vi "VsEP I-O Config.vi"(0 "Params":T1 {"STIMULUS"."dB STEPSIZE" format="%#_3g"; "STIMULUS"."START dB re 1g/ms" step=5}, 9 "Expt State":T6) -> (2 "Expt State out":T6, 3 "Datafile path":path, 4 "Runtime":T5, 6 "hidden out":T3, 10 "Max SPL":dbl, 14 "Analysis":T4, 15 "error out":errorcluster)   [LabVIEW 2020]
uses:
  CFTS Main Panel SubVIs/CFTS-Experiment State.ctl
  Typedefs/VsEP-Runtime Data.ctl
  Typedefs/VsEP-Hidden Params.ctl
  epl-vi-lib/Signal Synthesis VIs/Controls/Gate XCtl/Gate Control.xctl
  Typedefs/VsEP-Analysis State.ctl
  Typedefs/VsEP-Parameters.ctl
  Typedefs/VsEP-Stimulus Control.ctl
  epl-vi-lib/Connection VIs/Type Defs/Input sources.ctl
  epl-vi-lib/Connection VIs/Type Defs/Output sources.ctl
panel:
  out "num SPLs":i32
  in  "error in (no error)":errorcluster
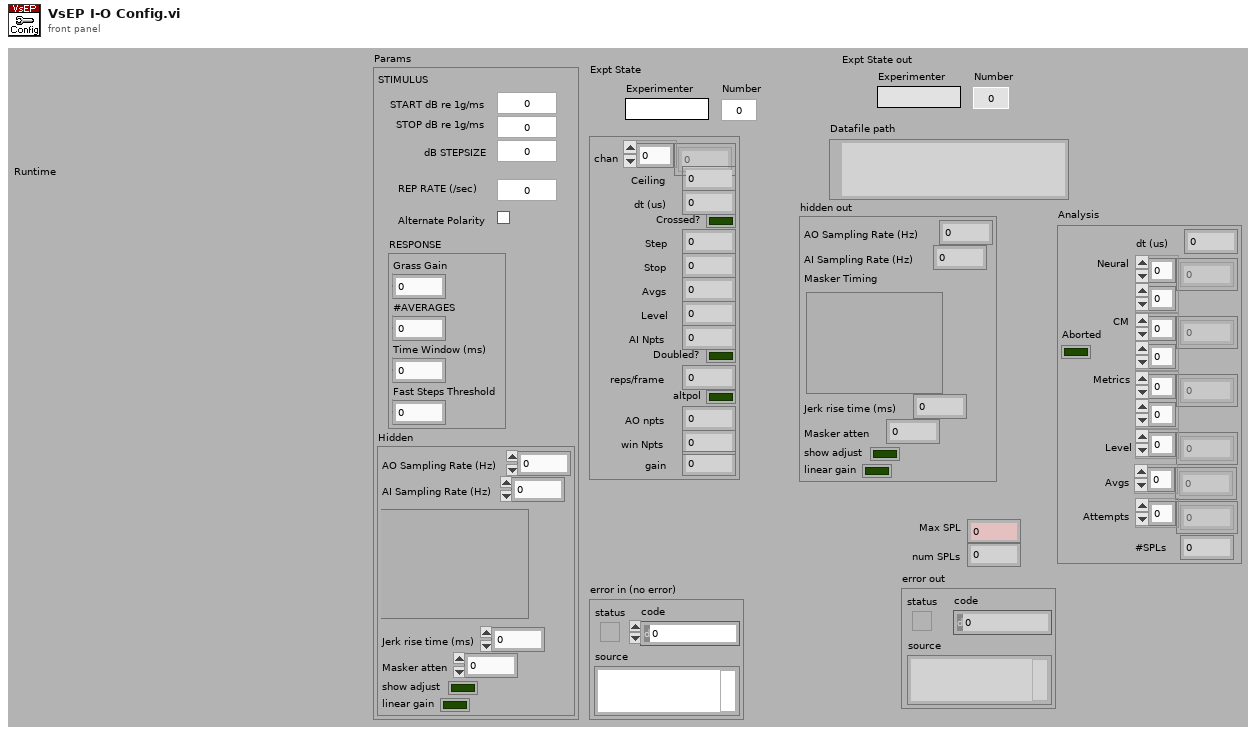
[diagram p1: front panel]
types:
  T1 = typedef "VsEP-Parameters.ctl" = cluster{"STIMULUS":T2, "RESPONSE":cluster{"Grass Gain":i32, "#AVERAGES":i32, "Time Window (ms)":sgl, "Fast Steps Threshold":i32}, "Hidden":T3}
  T2 = typedef "VsEP-Stimulus Control.ctl" = cluster{"START dB re 1g/ms":i32, "STOP dB re 1g/ms":i32, "dB STEPSIZE":sgl, "REP RATE (/sec)":dbl, "Alternate Polarity":bool, "Sampling Rate (Hz)":dbl}
  T3 = typedef "VsEP-Hidden Params.ctl" = cluster{"AO Sampling Rate (Hz)":dbl, "AI Sampling Rate (Hz)":dbl, "Masker Timing":cluster{"Active":bool, "Delay (ms)":dbl, "Width (ms)":dbl, "Ramp (ms)":dbl}, "Jerk rise time (ms)":dbl, "Masker atten":dbl, "show adjust":bool, "linear gain":bool}
  T4 = typedef "VsEP-Analysis State.ctl" = cluster{"dt (us)":dbl, "Neural":dbl[][], "CM":dbl[][], "Metrics":dbl[][], "Level":dbl[], "Avgs":i32[], "Attempts":i32[], "Aborted":bool, "#SPLs":i32}
  T5 = typedef "VsEP-Runtime Data.ctl" = cluster{"chan":i32[], "Ceiling":dbl, "dt (us)":dbl, "Crossed?":bool, "Step":dbl, "Stop":i32, "Avgs":i32, "Level":dbl, "AI Npts":i32, "Doubled?":bool, "reps/frame":i32, "altpol":bool, "AO npts":i32, "win Npts":i32, "gain":dbl}
  T6 = typedef "CFTS-Experiment State.ctl" = cluster{"Experimenter":string, "Number":u32, "Right":string, "Left":string, "Data Folder":path, "State File":path, "Version Info":string, "End Exposure Time":dbl, "Exposure Duration":string, "Run #":cluster{"CAP":i16, "ABR":i16, "DP":i16, "VsEP":i16, "MeasSeq":i16, "SubSeq":i16, "SFOAE":i16}}
  T7 = typedef "Output sources.ctl" = u16
  T8 = typedef "Input sources.ctl" = u16
  T9 = cluster{"Grass Gain":i32, "#AVERAGES":i32, "Time Window (ms)":sgl, "Fast Steps Threshold":i32}
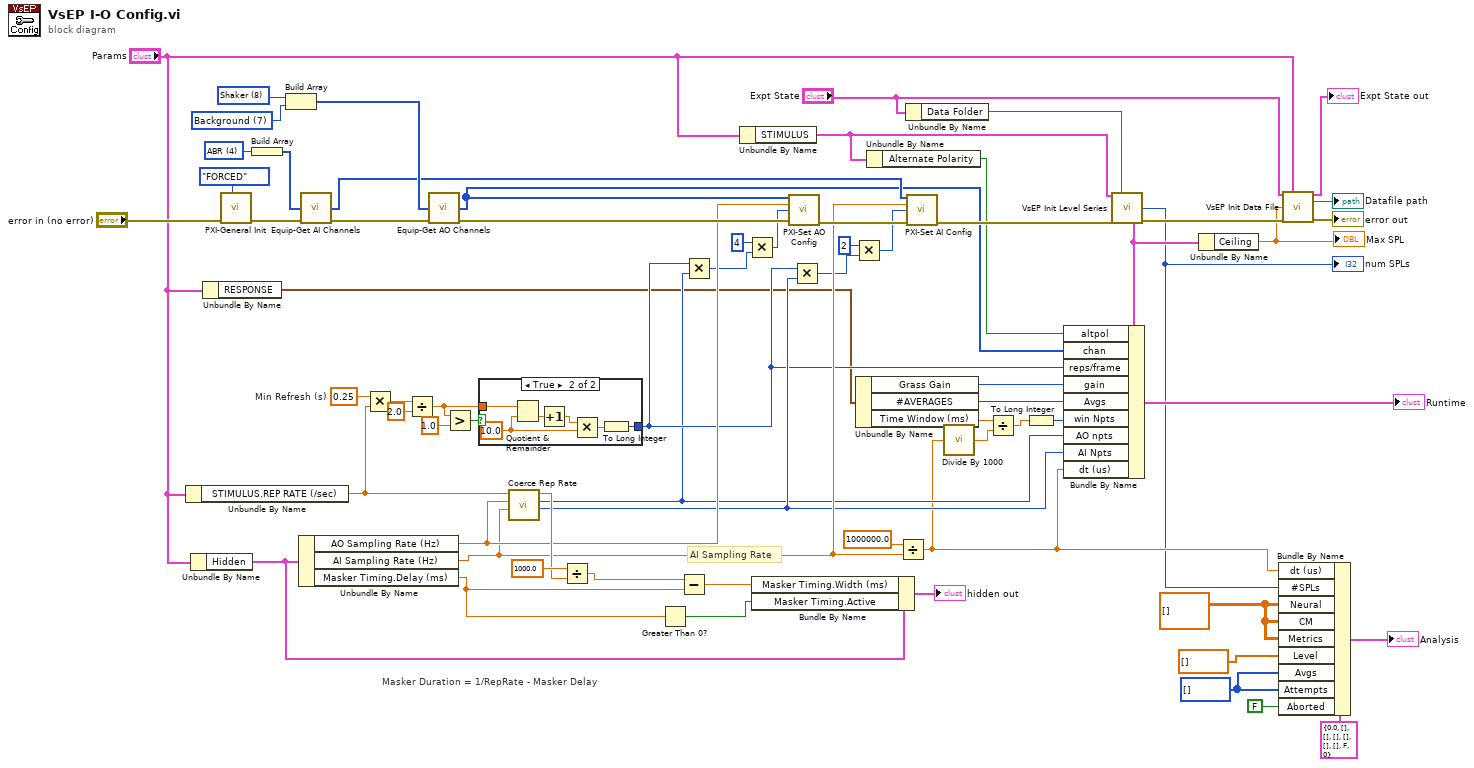
[diagram p0: block diagram]
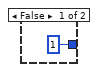
[diagram p2: hidden frame]
diagram:
  w12 = i32[] [] ("Avgs")
  w14 = dbl[][] [] ("Neural")
  w29 = 0.25  # Min Refresh (s)
  w55 = T7 7 items=["--unused--", "Right primary", "Right secondary", "Left primary", "Left secondary", "Shocks", "Startle", "Background"] ("Ring")
  w60 = T7 8 items=["--unused--", "Right primary", "Right secondary", "Left primary", "Left secondary", "Shocks", "Startle", "Background", "Shaker"] ("Ring")
  w64 = T8 4 items=["--unused--", "Probe Mic Right", "Probe Mic Left", "Cal Mic", "ABR", "CAP Right", "CAP Left", "Startle piezo", "Temperature", "Heart rate"] ("Ring")
  # "Masker Duration = 1/RepRate - Masker Delay"
  # "AI Sampling Rate"
  n1 = Unbundle By Name("Params") -> ("STIMULUS.REP RATE (/sec)"=w28:dbl)
  n2 = Unbundle By Name("Params") -> ("Hidden"=w4:T3)
  n3 = Unbundle By Name("Params") -> ("RESPONSE"=w5:T9)
  n4 = call "PXI-General Init.vi"("Double Buffer Mode"=enum32{"OFF", "ENABLED", "FORCED"}."FORCED", "error in (no error)"="error in (no error)") -> ("error out"=w62:errorcluster)  [unwired: 9 in]
  n5 = Build Array(w64) -> (w63:T8[])
  n6 = Build Array(w60, w55) -> (w61:T7[])
  n7 = Unbundle By Name(w4) -> ("AO Sampling Rate (Hz)"=w49:dbl, "AI Sampling Rate (Hz)"=w35:dbl, "Masker Timing.Delay (ms)"=w7:dbl)
  n8 = call "Equip-Get AI Channels.vi"("Inputs"=w63, "error in (no error)"=w62) -> ("AI Channels"=w45:i32[], "error out"=w46:errorcluster)  [unwired: 12 in]
  n9 = Multiply(x=w29, y=w28) -> (x*y=w30:dbl)
  n10 = Divide(x=w30, y=2.0) -> (x/y=w33:dbl)
  n11 = call "Equip-Get AO Channels.vi"("Outputs"=w61, "error in (no error)"=w46) -> ("AO Channels"=w24:i32[], "error out"=w51:errorcluster)  [unwired: 12 in]
  n12 = Greater?(x=w33, y=1.0) -> (0:w32:bool)
  n13 = case shown="True" w32 {
    tunnel: w33 -> [_ w75]
    tunnel: [1 w71] -> w23
    frame False {
    }
    frame True {
      w74 = 10.0 ("y")
      n14 = Quotient & Remainder(x=w75, y=w74) -> (floor(x/y)=w72:dbl)  [unwired: 1 out]
      n15 = Increment(x=w72) -> (x+1=w70:dbl)
      n16 = Multiply(x=w70, y=w74) -> (x*y=w73:dbl)
      n17 = To Long Integer(number=w73) -> (32bit integer=w71:i32)
    }
  }
  n18 = call "Coerce Rep Rate.vi"("AI sampling rate (Hz)"=w35, "AO sampling rate (Hz)"=w49, "Rep rate (Hz)"=w28) -> ("AI npts"=w25:i32, "AO npts"=w21:i32, "Coerced rep rate (Hz)"=w52:dbl)  [unwired: 5 in, 1 out]
  n19 = Divide(x=1000.0, y=w52) -> (x/y=w57:dbl)
  n20 = Greater Than 0?(x=w7) -> (x > 0?=w6:bool)
  n21 = Subtract(x=w57, y=w7) -> (x-y=w56:dbl)
  n22 = Multiply(x=w23, y=w21) -> (x*y=w27:i32)
  n23 = Unbundle By Name("Params") -> ("STIMULUS"=w3:T2)
  n24 = Multiply(x=4, y=w27) -> (x*y=w50:i32)
  n25 = Bundle By Name(cluster=w4, "Masker Timing.Width (ms)"=w56, "Masker Timing.Active"=w6) -> (→"hidden out":T3)
  n26 = call "PXI-Set AO Config.vi"("AO Channels"=w24, "Sampling Rate (Hz)"=w49, "Buffer Size"=w50, "error in (no error)"=w51) -> ("error out"=w48:errorcluster)  [unwired: 11 in]
  n27 = Multiply(x=w23, y=w25) -> (x*y=w26:i32)
  n28 = Multiply(x=2, y=w26) -> (x*y=w39:i32)
  n29 = Unbundle By Name(w5) -> ("Grass Gain"=w16:i32, "#AVERAGES"=w38:i32, "Time Window (ms)"=w20:sgl)
  n30 = Unbundle By Name(w3) -> ("Alternate Polarity"=w22:bool)
  n31 = Divide(x=1000000.0, y=w35) -> (x/y=w9:dbl)
  n32 = Unbundle By Name("Expt State") -> ("Data Folder"=w41:path)
  n33 = call "PXI-Set AI Config.vi"("AI Channels"=w45, "Sampling Rate (Hz)"=w35, "Buffer Size"=w39, "error in (no error)"=w48) -> ("error out"=w47:errorcluster)  [unwired: 11 in]
  n34 = call "Divide By 1000.vi"("X"=w9) -> ("X/1000"=w17:dbl)
  n35 = Divide(x=w20, y=w17) -> (x/y=w19:dbl)
  n36 = To Long Integer(number=w19) -> (32bit integer=w18:i32)
  n37 = call "VsEP Init Level Series.vi"("STIMULUS"=w3, "Data Folder"=w41, "error in (no error)"=w47) -> ("Max #Level"=w8:i32, "Runtime"=w36:T5, "error out"=w40:errorcluster)  [unwired: 10 in]
  "num SPLs" <- w8
  n38 = Bundle By Name(cluster=w36, "altpol"=w22, "chan"=w24, "reps/frame"=w23, "gain"=w16, "Avgs"=w38, "win Npts"=w18, "AO npts"=w21, "AI Npts"=w25, "dt (us)"=w9) -> (→"Runtime":T5)
  n39 = Unbundle By Name(w36) -> ("Ceiling"=w1:dbl)
  "Max SPL" <- w1
  n40 = Bundle By Name(cluster=T4 {"dt (us)"=0.0, "Neural"=[], "CM"=[], "Metrics"=[], "Level"=[], "Avgs"=[], "Attempts"=[], "Aborted"=FALSE, "#SPLs"=0} ("Analysis"), "dt (us)"=w9, "#SPLs"=w8, "Neural"=w14, "CM"=w14, "Metrics"=w14, "Level"=dbl[] [], "Avgs"=w12, "Attempts"=w12, "Aborted"=FALSE) -> (→"Analysis":T4)
  n41 = call "VsEP Init Data File.vi"("Expt State"="Expt State", "Params"="Params", "Max Jerk (dB re 1 g/ms)"=w1, "error in (no error)"=w40) -> ("Expt State out"=→"Expt State out":T6, "Datafile path"=→"Datafile path":path, "error out"=→"error out":errorcluster)  [unwired: 9 in]
